vi "Pump Action-Status Pump Start.vi"(8 "error in (no error)":errorcluster, 10 "Message Data":variant, 11 "Data Cluster in":T1 {"Pump Info"."Direction" items=["CW", "CCW"]; "Pump Info"."Speed" format="%03.0f"}) -> (0 "error out":errorcluster, 3 "Data Cluster out":T1 {"Pump Info"."Direction" items=["CW", "CCW"]; "Pump Info"."Speed" format="%03.0f"})   [LabVIEW 2020, in "Pump.lvlib"]
uses:
  Pump.lvlib
  Pump Hardware Configuration.ctl
  support/Message Queue/Message Cluster.ctl
  support/HW Message Cluster.ctl
  support/Message Queue/Message Queue.lvlib
  <instrlib>/WM Pump/WM Pump.lvlib
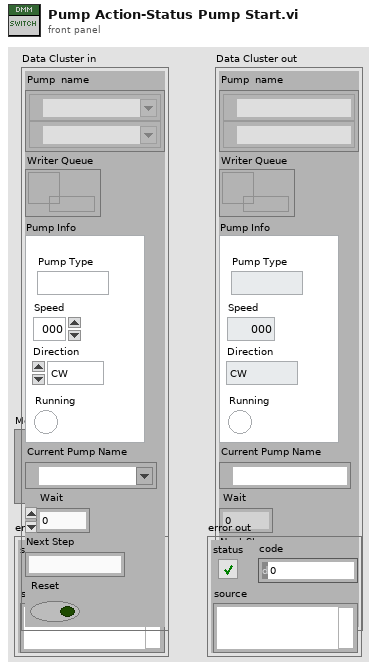
[diagram p1: front panel]
types:
  T1 = typedef "Pump.lvlib/Pump Hardware Configuration.ctl" = cluster{"Pump  name":refnum<visa-resource-name>[], "Writer Queue":refnum<queue>, "Pump Info":cluster{"Pump Type":string, "Speed":i32, "Direction":u16, "Running":bool}, "Current Pump Name":refnum<visa-resource-name>, "Wait":dbl, "Next Step":string, "Reset":bool}
  T2 = typedef "Message Queue.lvlib/HW Message Cluster.ctl" = cluster{"Writer Queue":refnum<queue>, "Writer Data":T3}
  T3 = typedef "Message Queue.lvlib/Message Cluster.ctl" = cluster{"Message":string, "Message Data":variant}
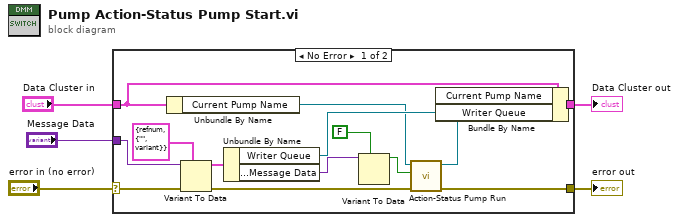
[diagram p0: block diagram]
diagram:
  n1 = case shown="No Error" "error in (no error)" {
    selector: "error in (no error)" -> [w15 w20]
    tunnel: "Message Data" -> [w14 _]
    tunnel: [w19 w21] -> w4
    tunnel: "Data Cluster in" -> [w18 w21]
    tunnel: [w7 w20] -> w2
    frame No Error {
      n2 = Unbundle By Name(w18) -> ("Current Pump Name"=w9:refnum<visa-resource-name>)
      n3 = Variant To Data(error in=w15, type=T2 {"Writer Queue"=refnum, "Writer Data"={"Message"="", "Message Data"=variant}}, Variant=w14) -> (data=w16:T2, error out=w6:errorcluster)
      n4 = Unbundle By Name(w16) -> ("Writer Queue"=w13:refnum<queue>, "Writer Data.Message Data"=w12:variant)
      n5 = Variant To Data(type=FALSE ("Backplane"), Variant=w12) -> (data=w10:bool)  [unwired: 1 in, 1 out]
      n6 = call <instrlib>:"Action-Status Pump Run.vi"("error in (no error)"=w6, "Start"=w10, "VISA resource name"=w9) -> ("error out"=w7:errorcluster, "VISA resource name out"=w8:refnum<visa-resource-name>)  [unwired: 7 in]
      n7 = Bundle By Name(cluster=w18, "Current Pump Name"=w8, "Writer Queue"=w13) -> (w19:T1)
    }
    frame Error {
    }
  }
  "Data Cluster out" <- w4
  "error out" <- w2
